vi "dynamicfindway.vi"(4 "new_x":dbl, 6 "pres_angle":dbl, 8 "angles":dbl[](array[numeric]), 9 "pres_y":dbl, 10 "distances":dbl[](array[numeric]), 11 "Numeric":i32) -> (0 "angleGoal":dbl, 1 "distanceGoal":cdb, 2 "pres_angle":dbl, 3 "repulsiveForce":cdb[](array[numeric]))   [LabVIEW 2015]
uses:
  <vilib>/imath/engines/lvmath2/RunTimeEngine/IndexRead/NIMS V(S).vi
  <instcachedir>/0/NIMS V(S)_0488751826AF41519A22953C041130DC.lvgen/NIMS V(S)_0488751826AF41519A22953C041130DC_000.vi
  <vilib>/imathl/engines/lvmath/Functions/Error Handling/Create Error.vi
  <vilib>/imath/engines/lvmath2/RunTimeEngine/BuiltInFunctions/max/2 inputs/NIMS_max(RG,RG)-no size check.vi
  <instcachedir>/0/NIMS_max(RG,RG)-no size check_F871939977644B7683C1350DCCAD7557.lvgen/NIMS_max(RG,RG)-no size check_F871939977644B7683C1350DCCAD7557_000.vi
  <vilib>/imath/engines/lvmath2/RunTimeEngine/BuiltInFunctions/atan2/NIMS_atan2.vi
  <instcachedir>/0/NIMS_atan2_A91AA4A7D42247EDBE8F76DB99AF04A4.lvgen/NIMS_atan2_A91AA4A7D42247EDBE8F76DB99AF04A4_002.vi
  <vilib>/imath/engines/lvmath2/RunTimeEngine/ArithmeticOperatorToken/NIMS_ArithmeticOperator_power(S).vi
  <instcachedir>/0/NIMS_ArithmeticOperator_power(S)_DFB67823F1414E5097C86E39787D8CA8.lvgen/NIMS_ArithmeticOperator_power(S)_DFB67823F1414E5097C86E39787D8CA8_014.vi
  <vilib>/imath/engines/lvmath2/RunTimeEngine/ErrorHandling/NIMS_Create Error From Enums.vi
  <vilib>/imath/engines/lvmath2/RunTimeEngine/NodeEndStatement/NIMS_NodeEndStatement_Output.vi
  <instcachedir>/0/NIMS_NodeEndStatement_Output_53EC0D466D134D7ABD903AC30B43404B.lvgen/NIMS_NodeEndStatement_Output_53EC0D466D134D7ABD903AC30B43404B_000.vi
  <instcachedir>/0/NIMS_NodeEndStatement_Output_53EC0D466D134D7ABD903AC30B43404B.lvgen/NIMS_NodeEndStatement_Output_53EC0D466D134D7ABD903AC30B43404B_001.vi
  <instcachedir>/0/NIMS_NodeEndStatement_Output_53EC0D466D134D7ABD903AC30B43404B.lvgen/NIMS_NodeEndStatement_Output_53EC0D466D134D7ABD903AC30B43404B_009.vi
  <vilib>/imath/engines/lvmath2/RunTimeEngine/ErrorHandling/NIMS_Finalize Error.vi
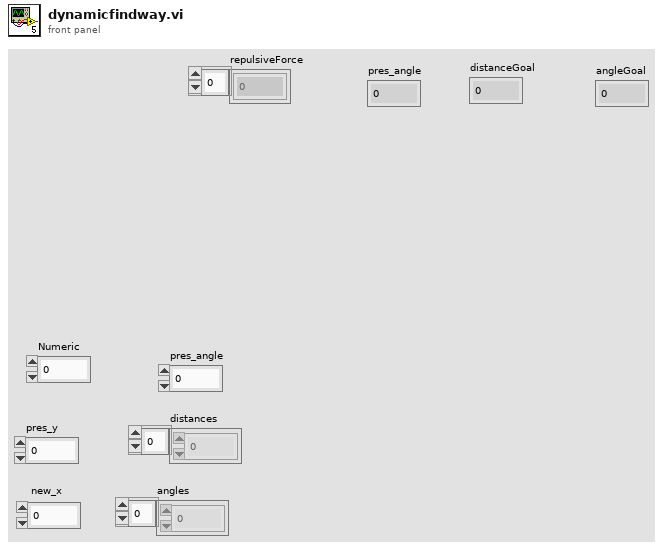
[diagram p1: front panel]
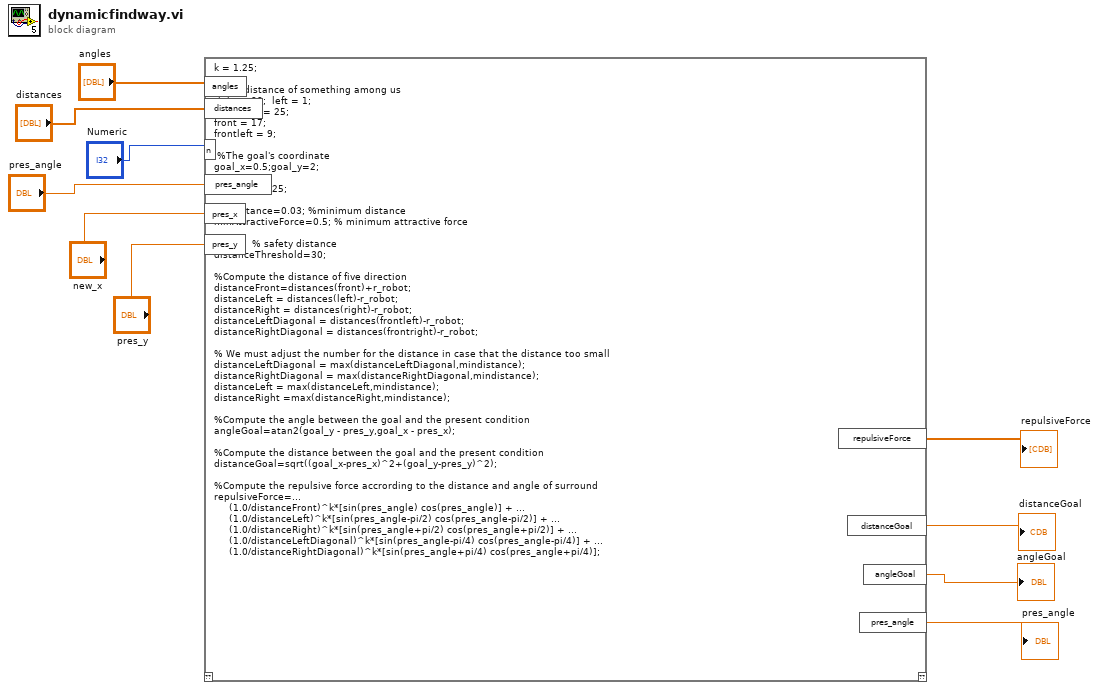
[diagram p0: block diagram]
diagram:
  n1 = mathscript code="k = 1.25; \n\n%The distance of something among us\nright = 33;  left = 1;  \nfrontright = 25;\nfront = 17;\nfrontleft = 9;\n\n %The goal's coordinate\ngoal_x=0.5;goal_y=2;  \n\nr_robot = 0.25;\n\nmindistance=0.03; %minimum distance\nminAttractiveForce=0.5; % minimum attractive force\n\nS=14;   % safety distance\ndistanceThreshold=30;\n\n%Compute the distance of five direction\ndistanceFront=distances(front)+r_robot;\ndistanceLeft = distances(left)-r_robot;\ndistanceRight = distances(right)-r_robot;\ndistanceLeftDiagonal = distances(frontleft)-r_robot;\ndistanceRightDiagonal = distances(frontright)-r_robot;\n\n% We must adjust the number for the distance in case that the distance too small\ndistanceLeftDiagonal = max(distanceLeftDiagonal,mindistance);\ndistanceRightDiagonal = max(distanceRightDiagonal,mindistance);\ndistanceLeft = max(distanceLeft,mindistance);\ndistanceRight =max(distanceRight,mindistance);\n\n%Compute the angle between the goal and the present condition\nangleGoal=atan2(goal_y - pres_y,goal_x - pres_x);\n\n%Compute the distance between the goal and the present condition\ndistanceGoal=sqrt((goal_x-pres_x)^2+(goal_y-pres_y)^2);\n\n%Compute the repulsive force accrording to the distance and angle of surround\nrepulsiveForce=...\n     (1.0/distanceFront)^k*[sin(pres_angle) cos(pres_angle)] + ...\n     (1.0/distanceLeft)^k*[sin(pres_angle-pi/2) cos(pres_angle-pi/2)] + ...\n     (1.0/distanceRight)^k*[sin(pres_angle+pi/2) cos(pres_angle+pi/2)] + ...\n     (1.0/distanceLeftDiagonal)^k*[sin(pres_angle-pi/4) cos(pres_angle-pi/4)] + ...\n     (1.0/distanceRightDiagonal)^k*[sin(pres_angle+pi/4) cos(pres_angle+pi/4)];"("n"="Numeric", "distances"="distances", "angles"="angles", "pres_angle"="pres_angle", "pres_x"="new_x", "pres_y"="pres_y") -> ("distanceGoal"=→"distanceGoal":cdb, "angleGoal"=→"angleGoal":dbl, "pres_angle"=→"pres_angle":dbl, "repulsiveForce"=→"repulsiveForce":cdb[])  [unwired: 1 in, 1 out]
